vi "RabbitMQPythonScaffold.vi"() -> ()   [LabVIEW 2019]
uses:
  API/config.ctl
  <vilib>/Platform/TimedLoop/XDataNode/timing_clust.ctl
  <vilib>/Platform/TimedLoop/XDataNode/nitl_modes.ctl
  <vilib>/Platform/TimedLoop/XDataNode/wakeup.ctl
  <vilib>/platform/TimedLoop/XDataNode/XDataNode.xnode
  rabbitmq.lvlib
  <vilib>/Platform/TimedLoop/XDataNode/XDNodeRunTimeDep.lvlib
panel:
  out "x != 0?":bool
  out "Received Messages":string[](array[string])
  out "Last Received Batch":string[](array[string])
  out "Sent Messages":string[](array[string])
  out "Last Sent Message":string
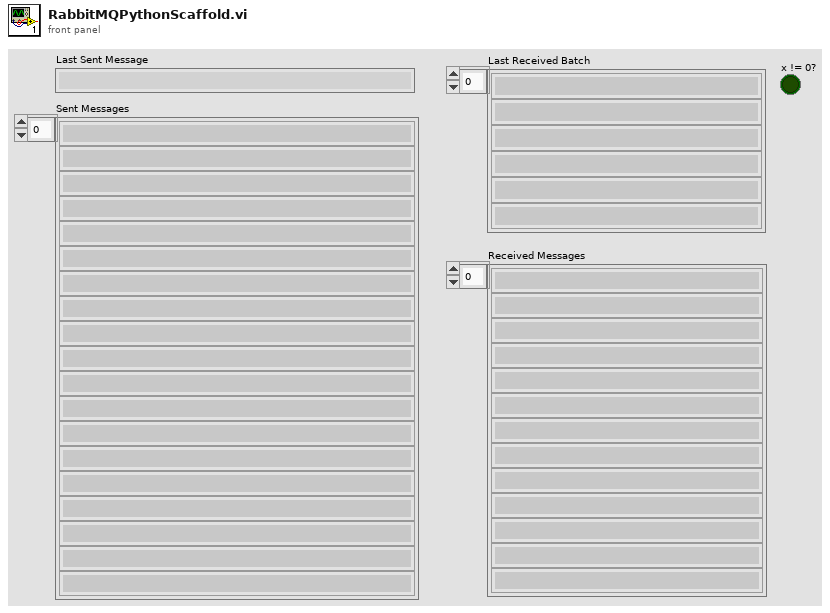
[diagram p1: front panel]
types:
  T1 = typedef "rabbitmq.lvlib/config.ctl" = cluster{"host":string, "port":i32, "virtual_host":string, "username":string, "password":string}
  T2 = typedef "rabbitmq.lvlib/session.ctl" = cluster{"script_path":path, "python_session":refnum<k35>}
  T3 = typedef "XDNodeRunTimeDep.lvlib/timing_clust.ctl" = cluster{"Expected End [f-1]":u64, "Actual End [f-1]":u64, "Finished Late? [f-1]":bool, "Expected End [i-1]":u64, "Actual End [i-1]":u64, "Finished Late? [i-1]":bool, "Expected Start [i]":u64, "Actual Start [i]":u64, "Expected Start [f]":u64, "Actual Start [f]":u64, "Source Name":string, "Structure Name":string, "Period":i64, "Deadline":i64, "Offset":i64, "Start":i64, "Priority":i32, "Timeout":i32, "Mode":T4, "Wakeup Reason":T5, "Error":errorcluster, "Source Type":string, "Secondary Source Type":string, "Global End Time":u64, "Global Start Time":u64, "Frame Duration":u64, "Iteration Duration":u64, "Assigned CPU":i32, "I/O Scan Engine Mode":u32}
  T4 = typedef "XDNodeRunTimeDep.lvlib/nitl_modes.ctl" = enum32{"No Change", "Process missed periods, maintain original phase", "Discard missed periods, maintain original phase", "Process missed periods, ignore original phase", "Discard missed periods, ignore original phase"}
  T5 = typedef "XDNodeRunTimeDep.lvlib/wakeup.ctl" = enum32{"Normal", "Aborted", "Asynchronous wakeup", "Timing source error", "Timed loop error", "Timeout"}
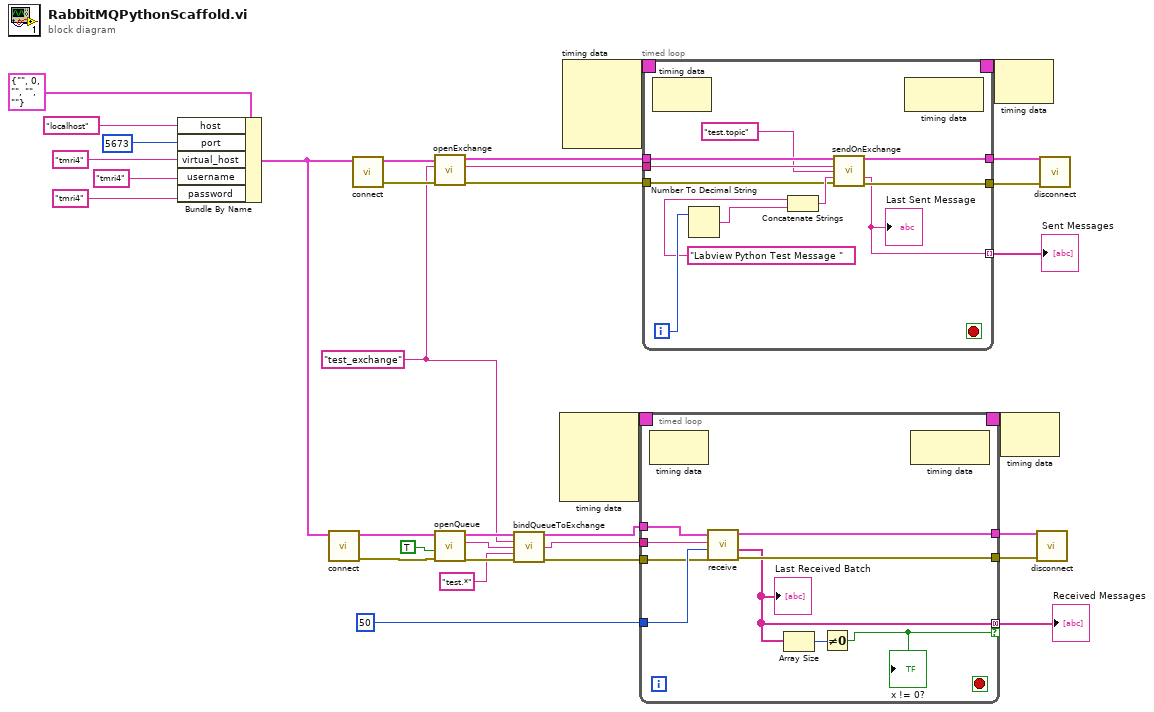
[diagram p0: block diagram]
diagram:
  w2 = "test_exchange"
  n1 = Bundle By Name(cluster=T1 {"host"="", "port"=0, "virtual_host"="", "username"="", "password"=""} ("Cluster"), "host"="localhost", "port"=5673, "virtual_host"="tmri4", "username"="tmri4", "password"="tmri4") -> (w23:T1)
  n2 = call "connect.vi"("RabbitMQ Config"=w23) -> ("error out"=w9:errorcluster, "RabbitMQ Session Out"=w10:T2)  [unwired: 9 in]
  n3 = call "connect.vi"("RabbitMQ Config"=w23) -> ("error out"=w15:errorcluster, "RabbitMQ Session Out"=w14:T2)  [unwired: 9 in]
  n4 = call "openExchange.vi"("error in (no error)"=w15, "Exchange Name In"=w2, "RabbitMQ Session In"=w14) -> ("error out"=w12:errorcluster, "Exchange Name out"=w11:string, "RabbitMQ Session Out"=w13:T2)  [unwired: 6 in]
  n5 = call "openQueue.vi"("error in (no error)"=w9, "Exclusive"=TRUE, "RabbitMQ Session In"=w10) -> ("error out"=w4:errorcluster, "Queue Name out"=w6:string, "RabbitMQ Session Out"=w8:T2)  [unwired: 6 in]
  n6 = call "bindQueueToExchange.vi"("RabbitMQ Session In"=w8, "Exchange Name In"=w2, "Queue Name In"=w6, "Routing Key In"="test.*", "error in (no error)"=w4) -> ("RabbitMQ Session Out"=w7:T2, "Queue Name out"=w5:string, "error out"=w3:errorcluster)  [unwired: 6 in, 2 out]
  n7 = node-c288() -> (w22:T3)  [unwired: 4 in]
  n8 = node-c288() -> (w28:T3)  [unwired: 4 in]
  n9 = timed-loop {
    timing: w22 -> [_]
    timing-out: [_] -> w21
    tunnel: [w43] -> w20
    tunnel: [w42] -> w19
    tunnel: w5 -> [w41]
    tunnel: [w39] -> w18 mode=concatenating if=w38
    tunnel: 50 ("Batch Size In") -> [w37]
    tunnel: w7 -> [w36]
    tunnel: w3 -> [w35]
    stop <- _ stop-if-true
    n10 = node-c288() -> ()  [unwired: 1 in, 1 out]
    n11 = call "receive.vi"("error in (no error)"=w35, "Batch Size In"=w37, "Queue Name in"=w41, "RabbitMQ Session In"=w36) -> ("error out"=w42:errorcluster, "Message Array"=w39:string[], "RabbitMQ Session Out"=w43:T2)  [unwired: 4 in, 1 out]
    "Last Received Batch" <- w39
    n12 = Array Size(array=w39) -> (size(s)=w40:i32)
    n13 = Not Equal To 0?(x=w40) -> (x != 0?=w38:bool)
    "x != 0?" <- w38
    n14 = node-c288() -> ()  [unwired: 1 in, 1 out]
  }
  "Received Messages" <- w18
  n15 = timed-loop {
    timing: w28 -> [_]
    timing-out: [_] -> w27
    tunnel: [w56] -> w26
    tunnel: [w55] -> w25
    tunnel: [w50] -> w24 mode=indexing
    tunnel: w13 -> [w49]
    tunnel: w12 -> [w48]
    tunnel: w11 -> [w47]
    i -> [w54]
    stop <- _ stop-if-true
    n16 = node-c288() -> ()  [unwired: 1 in, 1 out]
    n17 = Number To Decimal String(number=w54) -> (decimal integer string=w52:string)  [unwired: 1 in]
    n18 = Concatenate Strings("Labview Python Test Message ", w52) -> (w53:string)
    n19 = call "sendOnExchange.vi"("RabbitMQ Session In"=w49, "Exchange Name in"=w47, "Routing Key in"="test.topic", "Message In"=w53, "error in (no error)"=w48) -> ("RabbitMQ Session Out"=w55:T2, "Message out"=w50:string, "error out"=w56:errorcluster)  [unwired: 6 in, 2 out]
    "Last Sent Message" <- w50
    n20 = node-c288() -> ()  [unwired: 1 in, 1 out]
  }
  "Sent Messages" <- w24
  n21 = node-c288(w27) -> ()  [unwired: 1 out]
  n22 = node-c288(w21) -> ()  [unwired: 1 out]
  n23 = call "disconnect.vi"("error in (no error)"=w19, "RabbitMQ Session In"=w20) -> ()  [unwired: 9 in, 1 out]
  n24 = call "disconnect.vi"("error in (no error)"=w26, "RabbitMQ Session In"=w25) -> ()  [unwired: 9 in, 1 out]
